vi "readAVI.vi"() -> ()   [LabVIEW 2010]
panel:
  in  "stop":bool
  out "Image Out":T1(plugin-control)
  in  "AVI Path":path
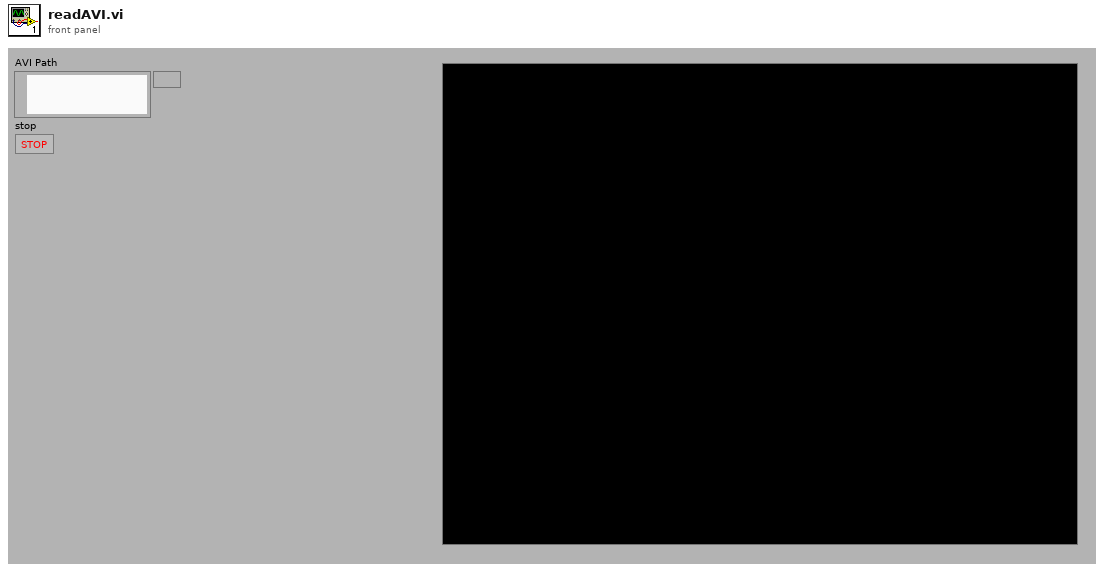
[diagram p1: front panel]
types:
  T1 = typedef "IMAQ Image.ctl" = refnum<image>
  T2 = typedef "AviRefnum.ctl" = refnum<k1>
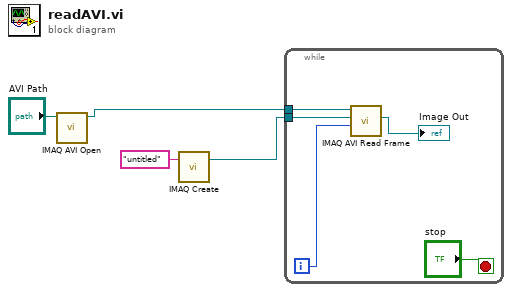
[diagram p0: block diagram]
diagram:
  n1 = call "IMAQ AVI Open"("AVI Path"="AVI Path") -> ("Avi Refnum"=w3:T2)  [unwired: 9 in, 1 out]
  n2 = call "IMAQ Create"("Image Name"="untitled") -> ("New Image"=w2:T1)  [unwired: 4 in, 1 out]
  n3 = while {
    tunnel: w3 -> [w9]
    tunnel: w2 -> [w8]
    i -> [w7]
    stop <- "stop" stop-if-true
    n4 = call "IMAQ AVI Read Frame"("Frame Number"=w7, "Image"=w8, "Avi Refnum"=w9) -> ("Image Out"=→"Image Out":T1)  [unwired: 5 in, 3 out]
  }
